vi "HovaCAL ppm.vi"(10 "Einheit MFC2 Eingang":T1, 11 "Eingangs Konzentration MFC2":dbl) -> (3 "Numerisch":dbl)   [LabVIEW 2020, in "EPA 1065.lvlib" / "HovaCAL Interference verificaton.lvlib"]
uses:
  HovaCAL Interference verificaton.lvlib
  Linearisierung V2/SpanEinstellungen/Einheit.ctl
  Linearisierung V2/SpanEinstellungen/SpanEinstellungen.lvlib
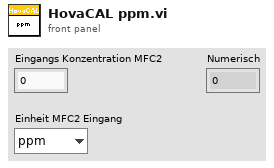
[diagram p1: front panel]
types:
  T1 = typedef "Linearisierung v2.lvlib/SpanEinstellungen.lvlib/Einheit.ctl" = enum16{"ppm", "%"}
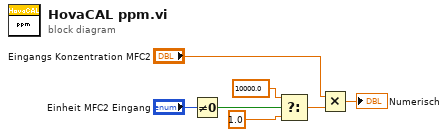
[diagram p0: block diagram]
diagram:
  n1 = Not Equal To 0?(x="Einheit MFC2 Eingang") -> (x != 0?=w2:bool)
  n2 = Select(t=10000.0, s=w2, f=1.0) -> (s? t:f=w4:dbl)
  n3 = Multiply(x="Eingangs Konzentration MFC2", y=w4) -> (x*y=→"Numerisch":dbl)
